vi "thermometers_display.vi"(11 "array type (2D Dbl)":dbl[](array[numeric])) -> (0 "Sensor 1":dbl(slide) scale=0.0..8.0, 1 "Sensor 6":dbl(slide) scale=0.0..8.0, 2 "Sensor 4":dbl(slide) scale=0.0..8.0, 3 "Sensor 8":dbl(slide) scale=0.0..8.0, 4 "Sensor 5":dbl(slide) scale=0.0..8.0, 5 "Sensor 2":dbl(slide) scale=0.0..8.0, 6 "Sensor 3":dbl(slide) scale=0.0..8.0, 7 "Sensor 7":dbl(slide) scale=0.0..8.0)   [LabVIEW 2021]
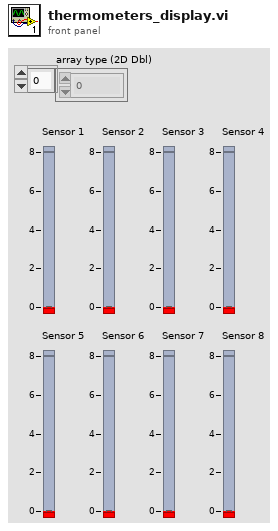
[diagram p1: front panel]
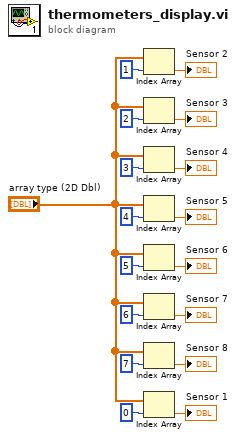
[diagram p0: block diagram]
diagram:
  n1 = Index Array(array="array type (2D Dbl)", index=1) -> (element=→"Sensor 2":dbl)
  n2 = Index Array(array="array type (2D Dbl)", index=2) -> (element=→"Sensor 3":dbl)
  n3 = Index Array(array="array type (2D Dbl)", index=3) -> (element=→"Sensor 4":dbl)
  n4 = Index Array(array="array type (2D Dbl)", index=4) -> (element=→"Sensor 5":dbl)
  n5 = Index Array(array="array type (2D Dbl)", index=5) -> (element=→"Sensor 6":dbl)
  n6 = Index Array(array="array type (2D Dbl)", index=6) -> (element=→"Sensor 7":dbl)
  n7 = Index Array(array="array type (2D Dbl)", index=7) -> (element=→"Sensor 8":dbl)
  n8 = Index Array(array="array type (2D Dbl)", index=0) -> (element=→"Sensor 1":dbl)
